vi "temp.vi"() -> ()   [LabVIEW 2014]
panel:
  in  "布尔":bool
  in  "字符串 3":string
  in  "字符串 2":string
  in  "字符串":string
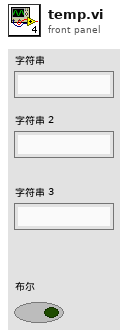
[diagram p1: front panel]
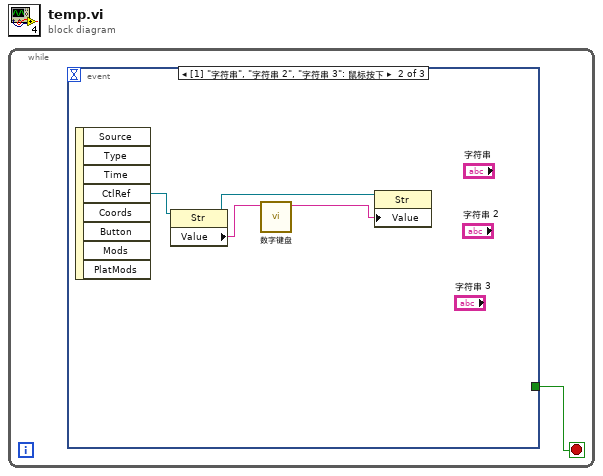
[diagram p0: block diagram]
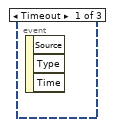
[diagram p2: hidden frame]
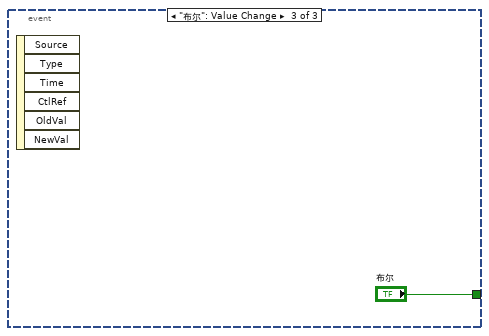
[diagram p3: hidden frame]
diagram:
  n1 = while {
    stop <- w1 stop-if-true
    n2 = event shown="[1] \"字符串\", \"字符串 2\", \"字符串 3\": 鼠标按下" {
      selector: _ -> [_ _ _]
      dyn-events: _ -> [_ _ _]
      timeout: _ -> [_ _ _]
      tunnel: [_ _ "布尔"] -> w1
      event Timeout {
        n3 = event-data() -> ()  [unwired: 1 in, 3 out]
      }
      event "字符串", "字符串 2", "字符串 3": Mouse Down {
        n4 = event-data() -> ("CtlRef"=w3:refnum<vi>)  [unwired: 1 in, 7 out]
        n5 = property class="Str"(reference=w3) -> (reference out=w2:refnum<vi>, "Value"=w4:string)  [unwired: 1 in, 1 out]
        n6 = call "数字键盘.vi"("数值输入"=w4) -> ("数值输出"=w5:string)  [unwired: 9 in, 1 out]
        n7 = property class="Str"(reference=w2, "Value"=w5) -> ()  [unwired: 1 in, 2 out]
      }
      event "布尔": Value Change {
        n8 = event-data() -> ()  [unwired: 1 in, 6 out]
      }
    }
  }
